vi "End Generation.vi"(10 "Num of elements":u32, 11 "Galvo signal readed":u32) -> (3 "End Generation":bool)   [LabVIEW 2015]
uses:
  <vilib>/rvi/Emulation/niFpgaSctlEmulationGetInTimedLoop.vi
  Globals/Global_Sample per Frame.vi
  <vilib>/rvi/Emulation/niFpgaProcessEmulError.vi
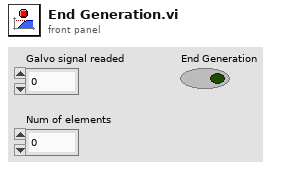
[diagram p1: front panel]
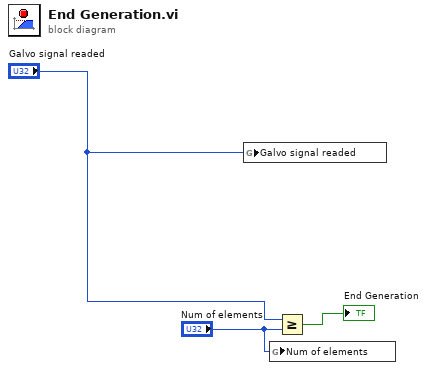
[diagram p0: block diagram]
diagram:
  n1 = global write "Global_Sample per Frame.vi" "Galvo signal readed"("Galvo signal readed") -> ()
  n2 = global write "Global_Sample per Frame.vi" "Num of elements"("Num of elements") -> ()
  n3 = Greater Or Equal?(x="Galvo signal readed", y="Num of elements") -> (x >= y?=→"End Generation":bool)
